vi "Scan Manager Core V5.vi"() -> ()   [LabVIEW 2015]
uses:
  <vilib>/Platform/TimedLoop/XDataNode/wakeup.ctl
  <vilib>/Platform/TimedLoop/XDataNode/XDNodeRunTimeDep.lvlib
  <vilib>/Platform/TimedLoop/XDataNode/nitl_modes.ctl
  <vilib>/Platform/TimedLoop/XDataNode/timing_clust.ctl
  <vilib>/Platform/TimedLoop/XDataNode/XDataNode.xnode
  Controls/FPGA Nain State.ctl
  LIDAR V2 Globals.vi
  <vilib>/eio/EIONode/EIONode.xnode
  <vilib>/rvi/DataTransferAndStorage/Container/XNode/niFpgaContainer.xnode
  <vilib>/rvi/eio/common/nirviEmuTemplateMethod_errors.vi
  <vilib>/rvi/FIFO/Fifo_Resource/nirvififoEmulationRead.vi
panel:
  in  "PFI2":bool
  in  "PFI3":bool
  in  "ActiveLedIndexDeb":u16
  in  "LedScanDebEn":bool
  out "Port0":u8 format="%.0b"
  out "Port1Bit4":bool
  out "Port1Bit5":bool
  out "Port1":u8 format="%.0b"
  in  "ScanMode":bool
  out "EnableSignal":bool
  in  "StopES":i16
  in  "StartES":i16
  in  "StartPulse":i16
  in  "StartAcq":i16
  in  "PulseEnd":bool
  out "PulseIndex":i16
  in  "WaitForPulseEndDelay":u8=3
  out "ActiveLedIndex":u16
  in  "SamplingEnable":bool
  in  "PulsePerLed":i16=199
  in  "SingleFrame":bool
  out "MainState":T1
  in  "NoOfLeds":u16=320
  in  "EndOfPulseGen":bool
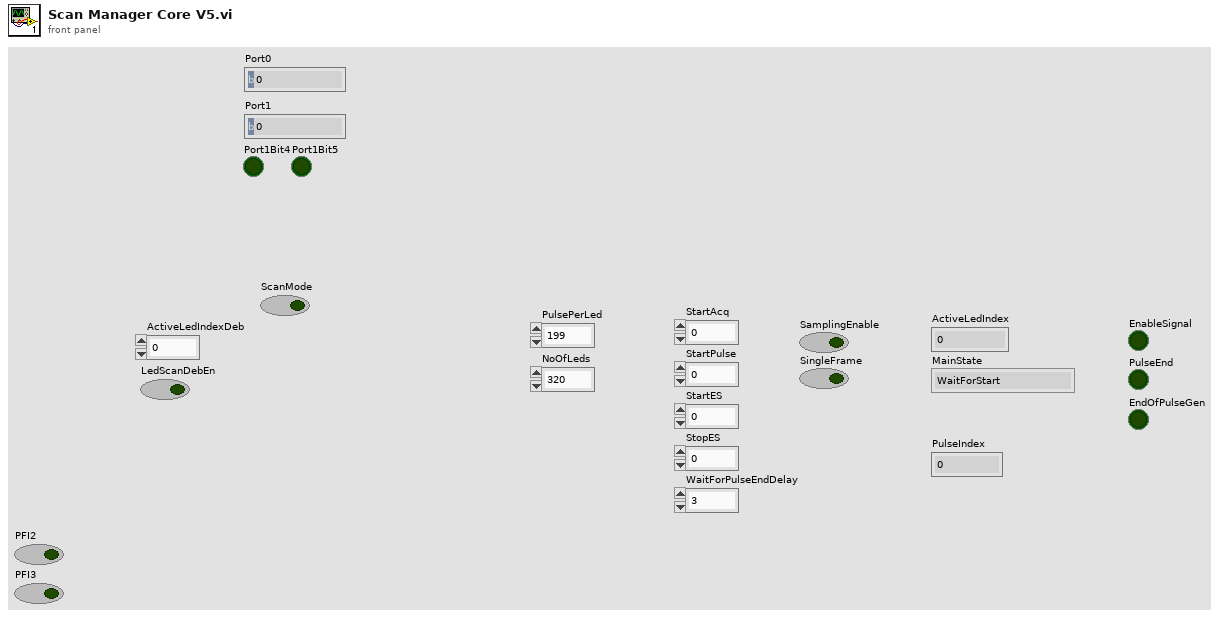
[diagram p1: front panel]
types:
  T1 = typedef "FPGA Nain State.ctl" = enum16{"WaitForStart", "SelectActiveLed", "WaitForNextPulse", "ActivatePulseCycle", "Error"}
  T2 = typedef "XDNodeRunTimeDep.lvlib/timing_clust.ctl" = cluster{"Expected End [f-1]":u64, "Actual End [f-1]":u64, "Finished Late? [f-1]":bool, "Expected End [i-1]":u64, "Actual End [i-1]":u64, "Finished Late? [i-1]":bool, "Expected Start [i]":u64, "Actual Start [i]":u64, "Expected Start [f]":u64, "Actual Start [f]":u64, "Source Name":string, "Structure Name":string, "Period":i64, "Deadline":i64, "Offset":i64, "Start":i64, "Priority":i32, "Timeout":i32, "Mode":T3, "Wakeup Reason":T4, "Error":errorcluster, "Source Type":string, "Secondary Source Type":string, "Global End Time":u64, "Global Start Time":u64, "Frame Duration":u64, "Iteration Duration":u64, "Assigned CPU":i32, "I/O Scan Engine Mode":u32}
  T3 = typedef "XDNodeRunTimeDep.lvlib/nitl_modes.ctl" = enum32{"No Change", "Process missed periods, maintain original phase", "Discard missed periods, maintain original phase", "Process missed periods, ignore original phase", "Discard missed periods, ignore original phase"}
  T4 = typedef "XDNodeRunTimeDep.lvlib/wakeup.ctl" = enum32{"Normal", "Aborted", "Asynchronous wakeup", "Timing source error", "Timed loop error", "Timeout"}
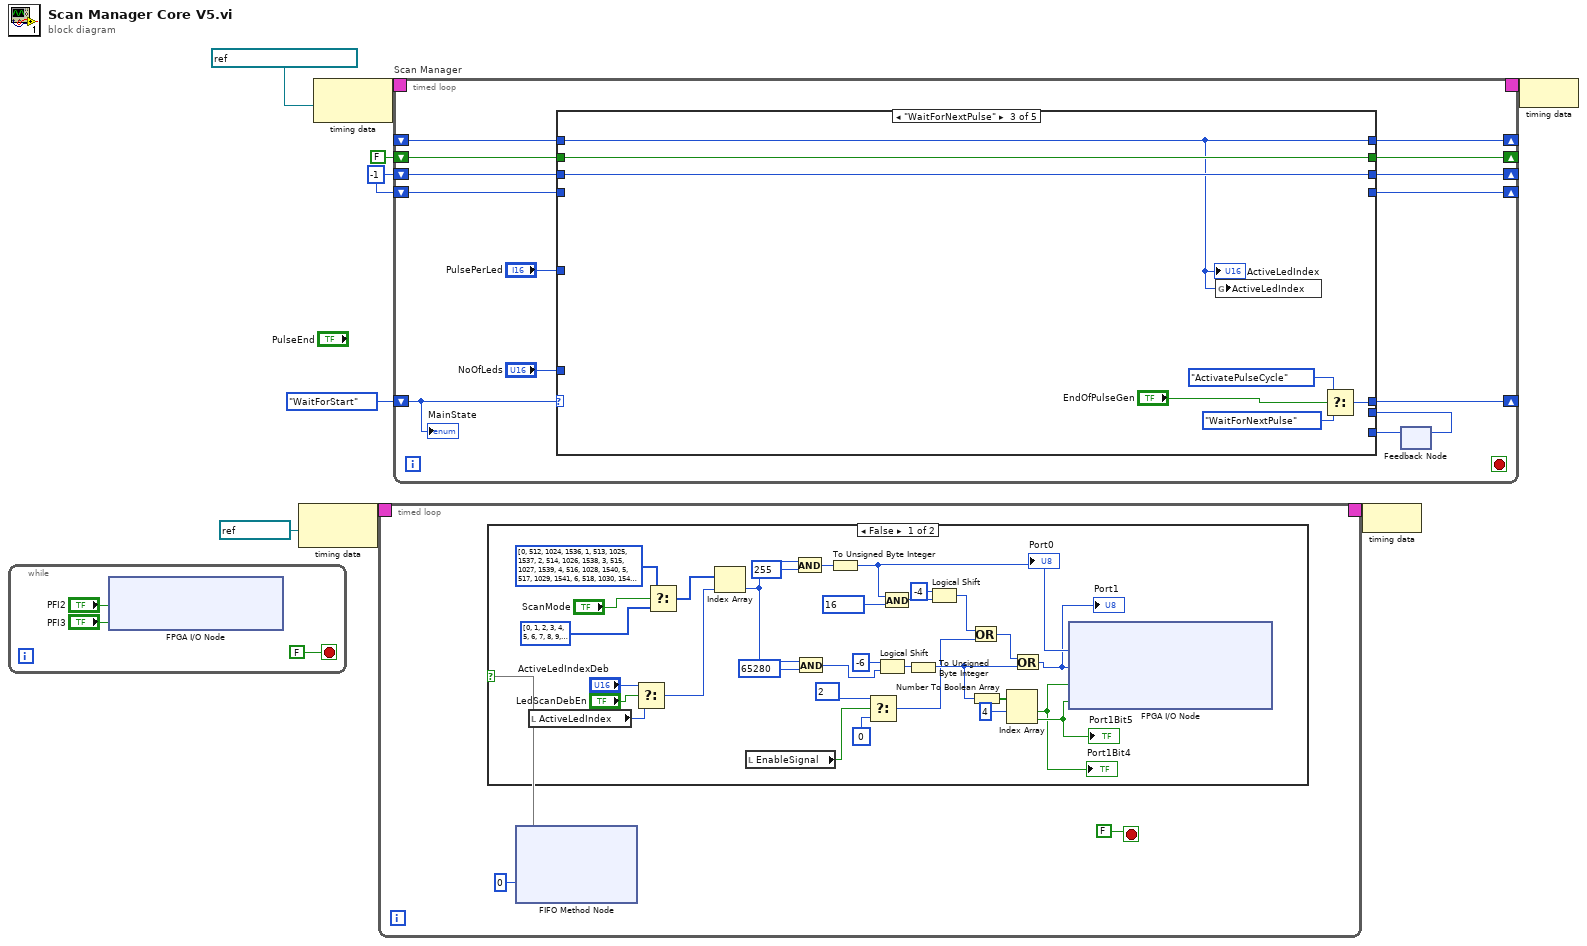
[diagram p0: block diagram]
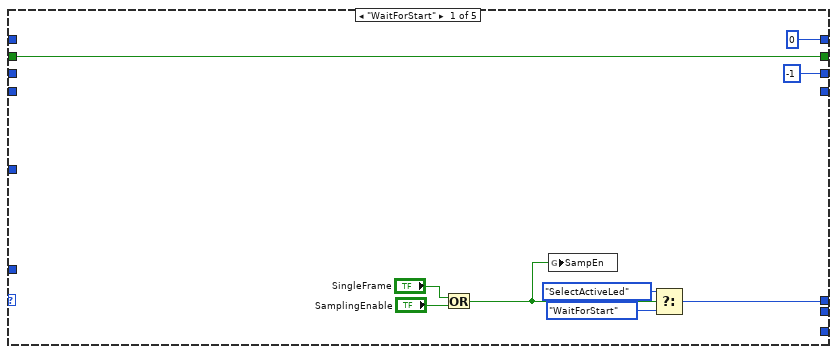
[diagram p3: hidden frame]
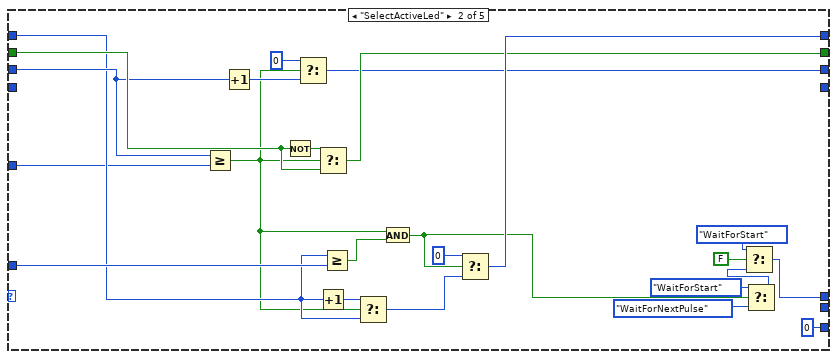
[diagram p4: hidden frame]
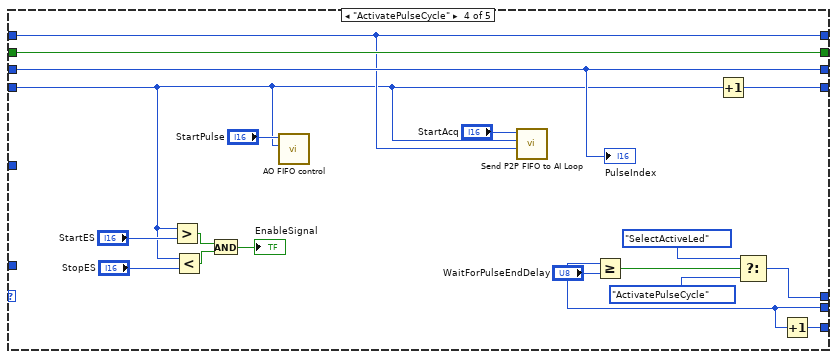
[diagram p5: hidden frame]
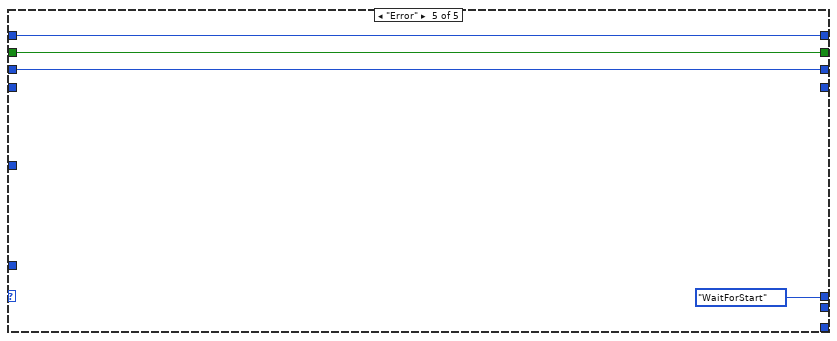
[diagram p6: hidden frame]
diagram:
  w5 = i16 -1
  n1 = while {
    stop <- FALSE stop-if-true
    n2 = xnode "FPGA I/O Node"("IO Module\\PFI 2 Wr Data"="PFI2", "IO Module\\PFI 3 Wr Data"="PFI3") -> ()  [unwired: 2 in, 2 out]
  }
  n3 = node-c288(refnum<k21> "130MHz" ("Source Name")) -> (w3:T2)
  n4 = node-c288(refnum<k21> "IO Module\\Data Clock" ("Source Name")) -> (w9:T2)
  n5 = timed-loop {
    timing: w3 -> [_]
    timing-out: [_] -> w2
    stop <- FALSE stop-if-true
    n6 = xnode ("FIFO Method Node")("Timeout"=0) -> ("Timed Out?"=w13)  [unwired: 1 in, 2 out]
    n7 = case shown="False" w13 {
      frame False {
        n8 = local read "ActiveLedIndex"() -> (w16:u16)
        n9 = Select(t="ActiveLedIndexDeb", s="LedScanDebEn", f=w16) -> (s? t:f=w28:u16)
        n10 = Select(t=u16[] [0, 512, 1024, 1536, 1, 513, 1025, 1537, 2, 514, 1026, 1538, 3, 515, 1027, 1539, 4, 516, 1028, 1540, 5, 517, 1029, 1541, 6, 518, 1030, 1542, 7, 519, 1031, 1543, 8, 520, 1032, 1544, 9, 521, 1033, 1545, 10, 522, 1034, 1546, 11, 523, 1035, 1547, 12, 524, 1036, 1548, 13, 525, 1037, 1549, 14, 526, 1038, 1550, 15, 527, 1039, 1551, 16, 528, 1040, 1552, 17, 529, 1041, 1553, 18, 530, 1042, 1554, 19, 531, 1043, 1555, 20, 532, 1044, 1556, 21, 533, 1045, 1557, 22, 534, 1046, 1558, 23, 535, 1047, 1559, 0, 0, 0, 0, 0, 0, 0, 0, 0, 0, 0, 0, 0, 0, 0, 0, 0, 0, 0, 0, 0, 0, 0, 0, 0, 0, 0, 0, 0, 0, 0, 0, 0, 0, 0, 0, 0, 0, 0, 0, 0, 0, 0, 0, 0, 0, 0, 0, 0, 0, 0, 0, 0, 0, 0, 0, 0, 0, 0, 0, 0, 0, 0, 0, 0, 0, 0, 0, 0, 0, 0, 0, 0, 0, 0, 0, 0, 0, 0, 0, 0, 0, 0, 0, 0, 0, 0, 0, 0, 0, 0, 0, 0, 0, 0, 0, 0, 0, 0, 0, 0, 0, 0, 0, 0, 0, 0, 0, 0, 0, 0, 0, 0, 0, 0, 0, 0, 0, 0, 0, 0, 0, 0, 0, 0, 0, 0, 0, 0, 0, 0, 0, 0, 0, 0, 0, 0, 0, 0, 0, 0, 0, 0, 0, 0, 0, 0, 0, 0, 0, 0, 0, 0, 0, 0, 0, 0, 0, 0, 0, 0, 0, 0, 0, 0, 0, 0, 0, 0, 0, 0, 0, 0, 0, 0, 0, 0, 0, 0, 0, 0, 0, 0, 0, 0, 0, 0, 0, 0, 0, 0, 0, 0, 0, 0, 0, 0, 0, 0, 0, 0, 0, 0, 0, 0, 0, 0, 0, 0, 0, 0, 0, 0, 0, 0, 0, 0, 0, 0, 0, 0, 0, 0, 0] ("Array"), s="ScanMode", f=u16[] [0, 1, 2, 3, 4, 5, 6, 7, 8, 9, 10, 11, 12, 13, 14, 15, 16, 17, 18, 19, 256, 257, 258, 259, 260, 261, 262, 263, 264, 265, 266, 267, 268, 269, 270, 271, 272, 273, 274, 275, 512, 513, 514, 515, 516, 517, 518, 519, 520, 521, 522, 523, 524, 525, 526, 527, 528, 529, 530, 531, 768, 769, 770, 771, 772, 773, 774, 775, 776, 777, 778, 779, 780, 781, 782, 783, 784, 785, 786, 787, 1024, 1025, 1026, 1027, 1028, 1029, 1030, 1031, 1032, 1033, 1034, 1035, 1036, 1037, 1038, 1039, 1040, 1041, 1042, 1043, 1280, 1281, 1282, 1283, 1284, 1285, 1286, 1287, 1288, 1289, 1290, 1291, 1292, 1293, 1294, 1295, 1296, 1297, 1298, 1299, 1536, 1537, 1538, 1539, 1540, 1541, 1542, 1543, 1544, 1545, 1546, 1547, 1548, 1549, 1550, 1551, 1552, 1553, 1554, 1555, 1792, 1793, 1794, 1795, 1796, 1797, 1798, 1799, 1800, 1801, 1802, 1803, 1804, 1805, 1806, 1807, 1808, 1809, 1810, 1811, 2048, 2049, 2050, 2051, 2052, 2053, 2054, 2055, 2056, 2057, 2058, 2059, 2060, 2061, 2062, 2063, 2064, 2065, 2066, 2067, 2304, 2305, 2306, 2307, 2308, 2309, 2310, 2311, 2312, 2313, 2314, 2315, 2316, 2317, 2318, 2319, 2320, 2321, 2322, 2323, 2560, 2561, 2562, 2563, 2564, 2565, 2566, 2567, 2568, 2569, 2570, 2571, 2572, 2573, 2574, 2575, 2576, 2577, 2578, 2579, 2816, 2817, 2818, 2819, 2820, 2821, 2822, 2823, 2824, 2825, 2826, 2827, 2828, 2829, 2830, 2831, 2832, 2833, 2834, 2835, 3072, 3073, 3074, 3075, 3076, 3077, 3078, 3079, 3080, 3081, 3082, 3083, 3084, 3085, 3086, 3087, 3088, 3089, 3090, 3091, 3328, 3329, 3330, 3331, 3332, 3333, 3334, 3335, 3336, 3337, 3338, 3339, 3340, 3341, 3342, 3343, 3344, 3345, 3346, 3347, 3584, 3585, 3586, 3587, 3588, 3589, 3590, 3591, 3592, 3593, 3594, 3595, 3596, 3597, 3598, 3599, 3600, 3601, 3602, 3603, 3840, 3841, 3842, 3843, 3844, 3845, 3846, 3847, 3848, 3849, 3850, 3851, 3852, 3853, 3854, 3855, 3856, 3857, 3858, 3859] ("Array")) -> (s? t:f=w19:u16[])
        n11 = Index Array(array=w19, index=w28) -> (element=w40:u16)
        n12 = local read "EnableSignal"() -> (w17:bool)
        n13 = And(x=w40, y=u16 255) -> (x .and. y?=w38:u16)
        n14 = And(x=w40, y=u16 65280) -> (x .and. y?=w37:u16)
        n15 = To Unsigned Byte Integer(number=w38) -> (unsigned 8bit integer=w34:u8)
        "Port0" <- w34
        n16 = Select(t=u8 2, s=w17, f=u8 0) -> (s? t:f=w23:u8)
        n17 = Logical Shift(y=i16 -6, x=w37) -> (x << y=w36:u16)
        n18 = And(x=w34, y=u8 16) -> (x .and. y?=w33:u8)
        n19 = To Unsigned Byte Integer(number=w36) -> (unsigned 8bit integer=w30:u8)
        n20 = Logical Shift(y=i16 -4, x=w33) -> (x << y=w26:u8)
        n21 = Or(x=w26, y=w23) -> (x .or. y?=w22:u8)
        n22 = Number To Boolean Array(number=w30) -> (Boolean array=w46:bool[])
        n23 = Index Array(array=w46, index #1=4 ("index")) -> (element #1=w31:bool, element #2=w44:bool)  [unwired: 1 in]
        "Port1Bit4" <- w31
        "Port1Bit5" <- w44
        n24 = Or(x=w22, y=w30) -> (x .or. y?=w29:u8)
        "Port1" <- w29
        n25 = xnode "FPGA I/O Node"("IO Module\\DIO Port 0 Wr Data"=w34, "IO Module\\DIO Port 1 Wr Data"=w29, "IO Module\\PFI 0 Wr Data"=w31, "IO Module\\PFI 1 Wr Data"=w44) -> ()  [unwired: 4 in, 4 out]
      }
      frame True {
      }
    }
  }
  n26 = timed-loop "Scan Manager" {
    timing: w9 -> [_]
    timing-out: [_] -> w8
    shift-right: [w61] -> _
    shift-left: FPGA_Nain_State."WaitForStart" ("MainState") -> [w62]
    shift-right: [w55] -> _
    shift-left: _ -> [w60]
    shift-right: [w57] -> _
    shift-left: FALSE -> [w59]
    shift-right: [w58] -> _
    shift-left: w5 -> [w56]
    shift-right: [w49] -> _
    shift-left: w5 -> [w50]
    stop <- _ stop-if-true
    n27 = feedback #1() -> (w52:u8)  [unwired: 1 in]
    n28 = case shown="\"WaitForNextPulse\"" w62 {
      tunnel: [w69 w92 w98 w114 FPGA_Nain_State."WaitForStart" ("MainState")] -> w61
      tunnel: [u16 0 ("ActiveLedIndex") w88 w97 w110 w125] -> w55
      tunnel: w60 -> [_ w80 w97 w110 w125]
      tunnel: [w66 w87 w102 w113 w124] -> w57
      tunnel: w59 -> [w66 w90 w102 w113 w124]
      tunnel: [i16 -1 ("t") w83 w101 w121 w123] -> w58
      tunnel: w56 -> [_ w86 w101 w121 w123]
      tunnel: "NoOfLeds" -> [_ w82 _ _ _]
      tunnel: [_ u8 0 _ w120 _] -> w53
      tunnel: w52 -> [_ _ _ w119 _]
      tunnel: "PulsePerLed" -> [_ w72 _ _ _]
      tunnel: w50 -> [_ _ _ w107 _]
      tunnel: [_ _ _ w112 _] -> w49
      frame "WaitForStart" {
        n29 = Or(x="SingleFrame", y="SamplingEnable") -> (x .or. y?=w63:bool)
        n30 = global write "LIDAR V2 Globals.vi" "SampEn"(w63) -> ()
        n31 = Select(t=FPGA_Nain_State."SelectActiveLed" ("MainState"), s=w63, f=FPGA_Nain_State."WaitForStart" ("MainState")) -> (s? t:f=w69:T1)
      }
      frame "SelectActiveLed" {
        n32 = Greater Or Equal?(x=w86, y=w72) -> (x >= y?=w75:bool)
        n33 = Increment(x=w86) -> (x+1=w85:i16)
        n34 = Not(x=w90) -> (.not. x?=w89:bool)
        n35 = Select(t=i16 0, s=w75, f=w85) -> (s? t:f=w83:i16)
        n36 = Select(t=w89, s=w75, f=w90) -> (s? t:f=w87:bool)
        n37 = Increment(x=w80) -> (x+1=w78:u16)
        n38 = Greater Or Equal?(x=w80, y=w82) -> (x >= y?=w76:bool)
        n39 = Select(t=w78, s=w75, f=w80) -> (s? t:f=w79:u16)
        n40 = And(x=w75, y=w76) -> (x .and. y?=w74:bool)
        n41 = Select(t=u16 0, s=w74, f=w79) -> (s? t:f=w88:u16)
        n42 = Select(t=FPGA_Nain_State."WaitForStart" ("MainState"), s=w74, f=FPGA_Nain_State."WaitForNextPulse" ("MainState")) -> (s? t:f=w93:T1)
        n43 = Select(t=FPGA_Nain_State."WaitForStart" ("MainState"), s=FALSE, f=w93) -> (s? t:f=w92:T1)
      }
      frame "WaitForNextPulse" {
        n44 = global write "LIDAR V2 Globals.vi" "ActiveLedIndex"(w97) -> ()
        n45 = Select(t=FPGA_Nain_State."ActivatePulseCycle" ("MainState"), s="EndOfPulseGen", f=FPGA_Nain_State."WaitForNextPulse" ("MainState")) -> (s? t:f=w98:T1)
        "ActiveLedIndex" <- w97
      }
      frame "ActivatePulseCycle" {
        n46 = Greater?(x=w107, y="StartES") -> (0:w104:bool)
        n47 = Less?(x=w107, y="StopES") -> (x < y?=w105:bool)
        n48 = And(x=w104, y=w105) -> (x .and. y?=→"EnableSignal":bool)
        n49 = call "AO FIFO control.vi"("Counter"=w107, "StartPulse"="StartPulse") -> ()  [unwired: 10 in]
        n50 = call "Send P2P FIFO to AI Loop.vi"("ActiveLedIndex"=w110, "TimingCounter"=w107, "StartAcq"="StartAcq") -> ()  [unwired: 9 in]
        n51 = Greater Or Equal?(x=w119, y="WaitForPulseEndDelay") -> (x >= y?=w117:bool)
        n52 = Increment(x=w107) -> (x+1=w112:i16)
        n53 = Select(t=FPGA_Nain_State."SelectActiveLed" ("MainState"), s=w117, f=FPGA_Nain_State."ActivatePulseCycle" ("MainState")) -> (s? t:f=w114:T1)
        n54 = Increment(x=w119) -> (x+1=w120:u8)
        "PulseIndex" <- w121
      }
      frame "Error" {
      }
    }
    n55 = feedback-in #1(w53) -> ()
    "MainState" <- w62
  }
  n56 = node-c288(w2) -> ()
  n57 = node-c288(w8) -> ()
